vi "Get Conditional Counts.vi"(1 "1D Array":u64[](array[numeric])) -> (15 "Conditional Counts":u64[][](array[numeric]), 17 "max value":u64, 19 "length":i32)   [LabVIEW 2014]
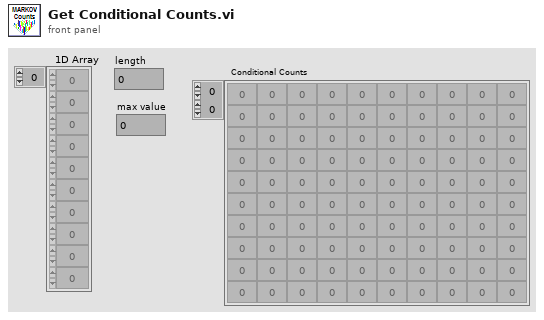
[diagram p1: front panel]
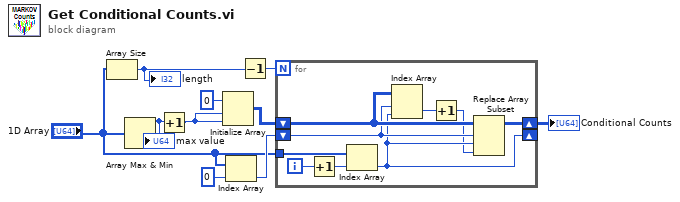
[diagram p0: block diagram]
diagram:
  n1 = Array Size(array="1D Array") -> (size(s)=w3:i32)
  "length" <- w3
  n2 = Array Max & Min(array="1D Array") -> (max value=w5:u64)  [unwired: 3 out]
  "max value" <- w5
  n3 = Increment(x=w5) -> (x+1=w6:u64)
  n4 = Initialize Array(u64 0 ("element"), w6, w6) -> (w9:u64[][])
  n5 = Index Array(array="1D Array", index=0) -> (element=w7:u64)
  n6 = Decrement(x=w3) -> (x-1=w2:i32)
  n7 = for {
    N: w2 -> [_]
    shift-right: [w13] -> w1
    shift-left: w9 -> [w17]
    shift-right: [w14] -> _
    shift-left: w7 -> [w16]
    tunnel: "1D Array" -> [w19]
    i -> [w18]
    n8 = Increment(x=w18) -> (x+1=w11:i32)
    n9 = Index Array(array=w19, index=w11) -> (element=w14:u64)
    n10 = Index Array(array=w17, index (row)=w16, index (col)=w14) -> (element=w15:u64)
    n11 = Increment(x=w15) -> (x+1=w12:u64)
    n12 = Replace Array Subset(array=w17, new element=w12, index (row)=w16, index (col)=w14) -> (w13:u64[][])
  }
  "Conditional Counts" <- w1
